vi "Run.vi"(6 "Type y_pred":T2(ring), 7 "Type y_true":T2(ring), 8 "error in (no error)":errorcluster caption="entrée d'erreur (pas d'erreur)", 9 "y_pred":string[][](array[string]), 10 "y_true":string[][](array[string]), 11 "Fbeta_Score.lvclass":refnum<class "Fbeta_Score.lvclass">) -> (0 "error out":errorcluster caption="sortie d'erreur", 2 "Data":T1, 3 "Fbeta_Score.lvclass":refnum<class "Fbeta_Score.lvclass">)   [LabVIEW 2020, in "Fbeta_Score.lvclass"]
doc: "Returns :\n\n- fbeta_score : float (if average is not None) or array of float, shape = [n_unique_labels]\nF-beta score of the positive class in binary classification or weighted average of the F-beta score of each class for the multiclass task."
uses:
  Fbeta_Score.lvclass
  Fbeta_Score.lvclass/Fbeta_Score.ctl
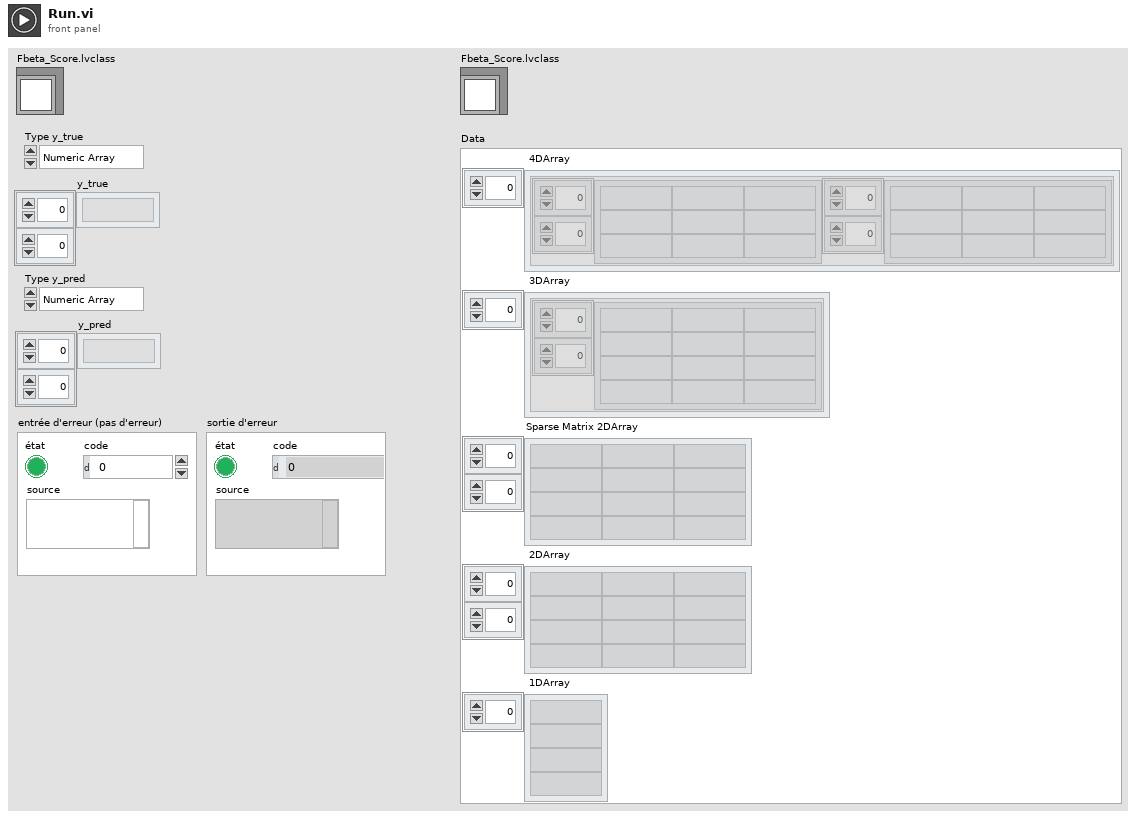
[diagram p1: front panel]
types:
  T1 = cluster{" 4DArray":cluster{"1":string[][], "2":string[][]}[], " 3DArray":cluster{"Tableau":string[][]}[], "Sparse Matrix 2DArray":string[][], " 2DArray":string[][], " 1DArray":string[]}
  T2 = enum16{"Numeric Array", "String Array", "Sparse"}
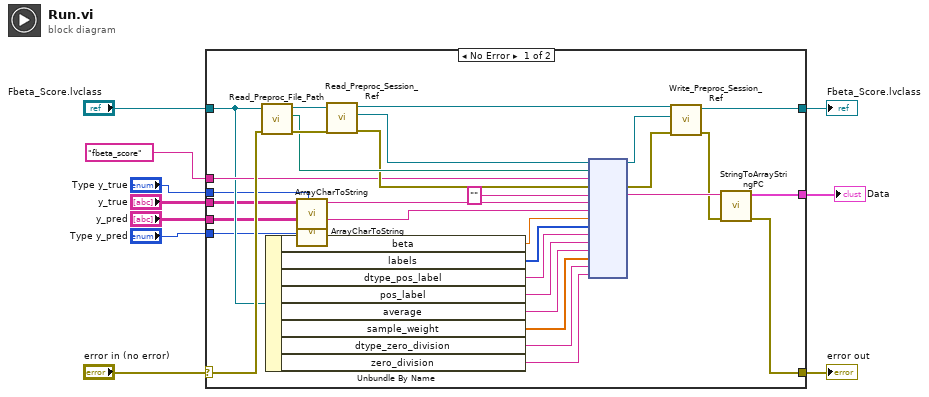
[diagram p0: block diagram]
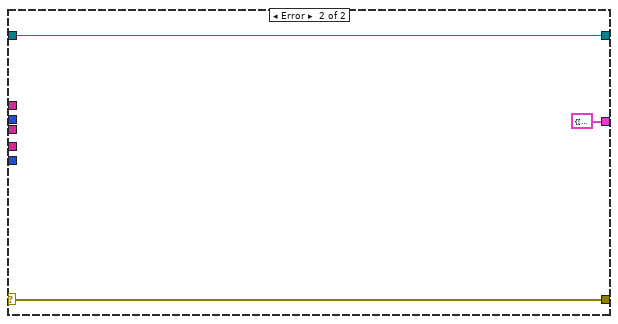
[diagram p2: hidden frame]
diagram:
  n1 = case shown="No Error" "error in (no error)" {
    selector: "error in (no error)" -> [w32 w44]
    tunnel: [w12 w44] -> w9
    tunnel: [w15 w43] -> w7
    tunnel: "Fbeta_Score.lvclass" -> [w30 w43]
    tunnel: "fbeta_score" -> [w31 _]
    tunnel: "y_true" -> [w21 _]
    tunnel: "y_pred" -> [w20 _]
    tunnel: "Type y_true" -> [w17 _]
    tunnel: "Type y_pred" -> [w16 _]
    tunnel: [w11 T1 {" 4DArray"=[], " 3DArray"=[], "Sparse Matrix 2DArray"=[], " 2DArray"=[], " 1DArray"=[]} ("Data")] -> w1
    frame No Error {
      n2 = call-dynamic "Read_Preproc_File_Path.vi"("error in (no error)"=w32, "Python in"=w30) -> ("error out"=w40:errorcluster, "File_Path"=w39:path, "Python out"=w41:refnum<class "Fbeta_Score.lvclass">)  [unwired: 7 in]
      n3 = Unbundle By Name(w30) -> ("beta"=w29:dbl, "labels"=w28:i32[], "dtype_pos_label"=w27:string, "pos_label"=w26:string, "average"=w25:string, "sample_weight"=w24:dbl[], "dtype_zero_division"=w23:string, "zero_division"=w22:string)
      n4 = call "ArrayCharToString.vi"("Type"=w17, "TAB"=w21) -> ("Instruction"=w19:string)  [unwired: 9 in]
      n5 = call "ArrayCharToString.vi"("Type"=w16, "TAB"=w20) -> ("Instruction"=w18:string)  [unwired: 9 in]
      n6 = call-dynamic "Read_Preproc_Session_Ref.vi"("error in (no error)"=w40, "Python in"=w41) -> ("error out"=w37:errorcluster, "Session_ref"=w38:refnum<k35>, "Python out"=w36:refnum<class "Fbeta_Score.lvclass">)  [unwired: 7 in]
      n7 = node(w38, w39, w31, w37, "", w19, w18, w29, w28, w27, w26, w25, w24, w23, w22) -> (w34:refnum<k35>, w35:errorcluster, w14:string)  [unwired: 10 in, 2 out]
      n8 = call-dynamic "Write_Preproc_Session_Ref.vi"("error in (no error)"=w35, "Session_ref"=w34, "Python in"=w36) -> ("error out"=w13:errorcluster, "Python out"=w15:refnum<class "Fbeta_Score.lvclass">)  [unwired: 7 in]
      n9 = call "StringToArrayStringPC.vi"("sortie d'erreur"=w13, "Return value"=w14) -> ("sortie d'erreur"=w12:errorcluster, "Data"=w11:T1)  [unwired: 8 in]
    }
    frame Error {
    }
  }
  "error out" <- w9
  "Fbeta_Score.lvclass" <- w7
  "Data" <- w1
